vi "Process.vi"(8 "error in":errorcluster, 11 "SynchiIO.PXI4461":refnum<class "SynchiIO.PXI4461.lvclass">) -> (0 "error out":errorcluster, 3 "SynchiIO.PXI4461 out":refnum<class "SynchiIO.PXI4461.lvclass">)   [LabVIEW 2016, in "SynchiIO.PXI4461.lvclass"]
doc: "---------------------------------------------------------------\nJKI State Machine Objects™\nhttp://jki.net/state-machine-objects/\nCopyright (C) 2005-2015, JKI <info@jki.net>\nALL RIGHTS RESERVEDJKI State Machine Objects (SMO) 1.0.0.5\nJKI - JKI\nCopyright (c) 2016, JKI"
uses:
  SynchiIO.PXI4461.lvclass
  <vilib>/JKI/JKI SMO/SMO/SMO.lvclass
  <vilib>/JKI/JKI SMO/SMO/Typedefs/Parent Call--Enum.ctl
  <resource>/objmgr/ni.dex.rc
  trunk/SynchIO/SynchIO.USB4431/SynchIO.USB4431.lvclass
  C:/Program Files (x86)/National Instruments/LabVIEW 2016/vi.lib/JKI/JKI SMO/SMO/SMO.lvclass
  I:/levy_SVN/lockin/branches/jlevy/SMO/trunk/SynchIO/SynchIO/SynchIO.lvclass
panel:
  in  "Start":bool
  in  "stop":bool
  out "State History":string
  out "Current State":string="Exit"
  in  "Tab Control":T1(tab)=enum."AO Config"
  in  "AI Configuration":T2(array[cluster])=[{"AI.Coupling"=enum."DC", "AI.Max"=10.0, "AI.Min"=-10.0, "Input physical channels"="Dev1/ai0:3"}]
  in  "AO Configuration":T3(array[cluster])=[{"Output physical channels"="Dev1/ao0", "AO. Max"=3.5, "AO.Min"=-3.5}]
  in  "sampling info":cluster{"Fs":dbl, "#s":dbl}={"Fs"=102388.0, "#s"=7876.0}
  in  "AI Buffer Size (S)":i32=100
  in  "error in 2":errorcluster
  out "error out 2":errorcluster
  in  "AO":T4={"AO amp (V)"=[1.0, 0.0, 0.0, 0.0, 0.0, 0.0, 0.0, 0.0], "AO DC (V)"=[0.0, 0.0, 0.0, 0.0, 0.0, 0.0, 0.0, 0.0], "AO f (Hz)"=[13.0, 13.0, 13.0, 13.0, 13.0, 13.0, 13.0, 13.0], "AO phi (deg)"=[0.0, 0.0, 0.0, 0.0, 0.0, 0.0, 0.0, 0.0], "function"=[enum."Sine Wave", enum."Sine Wave", enum."Sine Wave", enum."Sine Wave", enum."Sine Wave", enum."Sine Wave", enum."Sine Wave", enum."Sine Wave"]} {"AO DC (V)" format="%#_6p"; "AO amp (V)" format="%#_6p"}
  out "Signals Graph":waveform(dbl)[](graph)=[{"t0"=timestamp(3565974471.4961195 s since 1904-01-01), "dt"=1.0, "Y"=array[6023 elements], "attributes"=variant("NI_ChannelName"=variant(string "Dev2/ai0"), "NI_UnitDescription"=variant(string "Volts"))}, {"t0"=timestamp(3565974471.4961195 s since 1904-01-01), "dt"=1.0, "Y"=array[6023 elements], "attributes"=variant("NI_ChannelName"=variant(string "Dev2/ai1"), "NI_UnitDescription"=variant(string "Volts"))}, {"t0"=timestamp(3565974471.4961195 s since 1904-01-01), "dt"=1.0, "Y"=array[6023 elements], "attributes"=variant("NI_ChannelName"=variant(string "Dev2/ai2"), "NI_UnitDescription"=variant(string "Volts"))}, {"t0"=timestamp(3565974471.4961195 s since 1904-01-01), "dt"=1.0, "Y"=array[6023 elements], "attributes"=variant("NI_ChannelName"=variant(string "Dev2/ai3"), "NI_UnitDescription"=variant(string "Volts"))}, {"t0"=timestamp(3565974471.554943 s since 1904-01-01), "dt"=1.0, "Y"=array[6023 elements], "attributes"=variant("NI_ChannelName"=variant(string "Dev2/ai0"), "NI_UnitDescription"=variant(string "Volts"))}, {"t0"=timestamp(3565974471.554943 s since 1904-01-01), "dt"=1.0, "Y"=array[6023 elements], "attributes"=variant("NI_ChannelName"=variant(string "Dev2/ai1"), "NI_UnitDescription"=variant(string "Volts"))}]
  out "Signals Graph 2":waveform(dbl)[](graph)=[{"t0"=timestamp(3565974471.4961195 s since 1904-01-01), "dt"=1.0, "Y"=array[6023 elements], "attributes"=variant("NI_ChannelName"=variant(string "Dev2/ai0"), "NI_UnitDescription"=variant(string "Volts"))}, {"t0"=timestamp(3565974471.4961195 s since 1904-01-01), "dt"=1.0, "Y"=array[6023 elements], "attributes"=variant("NI_ChannelName"=variant(string "Dev2/ai1"), "NI_UnitDescription"=variant(string "Volts"))}, {"t0"=timestamp(3565974471.4961195 s since 1904-01-01), "dt"=1.0, "Y"=array[6023 elements], "attributes"=variant("NI_ChannelName"=variant(string "Dev2/ai2"), "NI_UnitDescription"=variant(string "Volts"))}, {"t0"=timestamp(3565974471.4961195 s since 1904-01-01), "dt"=1.0, "Y"=array[6023 elements], "attributes"=variant("NI_ChannelName"=variant(string "Dev2/ai3"), "NI_UnitDescription"=variant(string "Volts"))}, {"t0"=timestamp(3565974471.554943 s since 1904-01-01), "dt"=1.0, "Y"=array[6023 elements], "attributes"=variant("NI_ChannelName"=variant(string "Dev2/ai0"), "NI_UnitDescription"=variant(string "Volts"))}, {"t0"=timestamp(3565974471.554943 s since 1904-01-01), "dt"=1.0, "Y"=array[6023 elements], "attributes"=variant("NI_ChannelName"=variant(string "Dev2/ai1"), "NI_UnitDescription"=variant(string "Volts"))}]
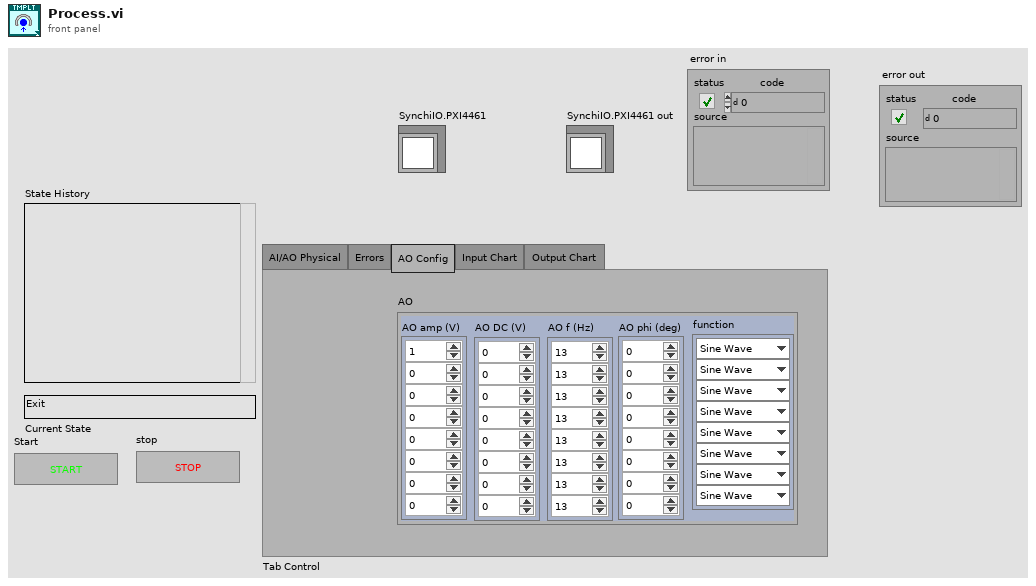
[diagram p1: front panel]
types:
  T1 = enum32{"AI/AO Physical", "Errors", "AO Config", "Input Chart", "Output Chart "}
  T2 = cluster{"AI.Coupling":enum16{"AC", "DC", "GND"}, "AI.Max":dbl, "AI.Min":dbl, "Input physical channels":tag}[]
  T3 = cluster{"Output physical channels":tag, "AO. Max":dbl, "AO.Min":dbl}[]
  T4 = cluster{"AO amp (V)":dbl[], "AO DC (V)":dbl[], "AO f (Hz)":dbl[], "AO phi (deg)":dbl[], "function":enum16{"Sine Wave", "Triangle Wave", "Square Wave", "Sawtooth Wave"}[]}
  T5 = typedef "SMO.lvclass/Parent Call--Enum.ctl" = enum16{"Allows parent to run", "Does not request parent to run"}
  T6 = enum32{"invalid app kind", "Development System", "Run Time System", "Student Edition", "Embedded LabVIEW", "Evaluation", "Custom"}
  T7 = enum32{"Invalid", "Standard", "Closed", "Hidden", "Minimized", "Maximized"}
  T8 = cluster{"Core":cluster{"Current VI Reference":refnum<vi>, "Close Panel on Exit?":bool, "error":errorcluster}, "Self Reference":refnum<class "SynchiIO.PXI4461.lvclass">, "Your string data":string, "AI Buffer Size (S)":i32, "AI Configuration":cluster{"AI.Coupling":enum16{"AC", "DC", "GND"}, "AI.Max":dbl, "AI.Min":dbl, "Input physical channels":tag}[], "AO Configuration":cluster{"Output physical channels":tag, "AO. Max":dbl, "AO.Min":dbl}[], "sampling info":cluster{"Fs":dbl, "#s":dbl}, "AI task":refnum<k21>[], "AO Task":refnum<k21>[], "AI Data":waveform(dbl)[], "AO Data":waveform(dbl)[], "AO":cluster{"AO amp (V)":dbl[], "AO DC (V)":dbl[], "AO f (Hz)":dbl[], "AO phi (deg)":dbl[], "function":enum16{"Sine Wave", "Triangle Wave", "Square Wave", "Sawtooth Wave"}[]}, "Iteration":i32, "writer endpoint":refnum<k21>, "reader endpoint":refnum<k21>, "url":string}
  T9 = cluster{"Current VI Reference":refnum<vi>, "Close Panel on Exit?":bool, "error":errorcluster}
  T10 = typedef "SynchIO.USB4431.lvclass/ProtectedEvents--Cluster.ctl" = cluster{"API_Template":refnum<user-event>}
  T11 = typedef "SynchiIO.PXI4461.lvclass/ProtectedEvents--Cluster.ctl" = cluster{"API_Template":refnum<user-event>}
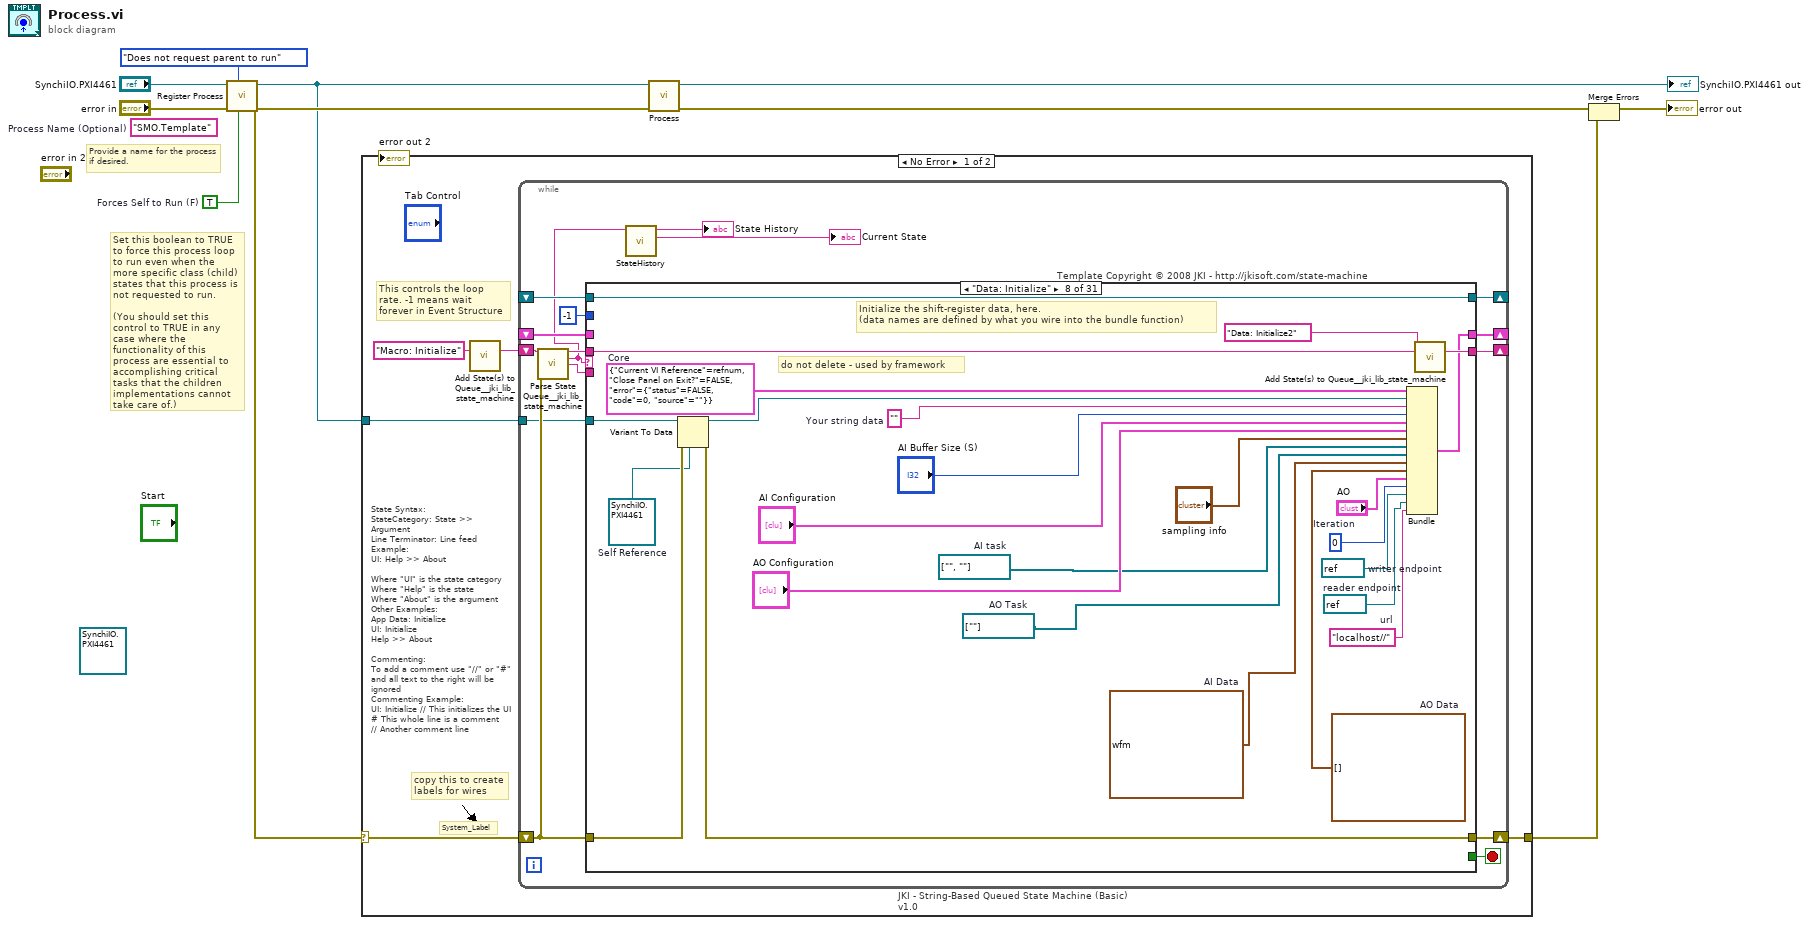
[diagram p0: block diagram]
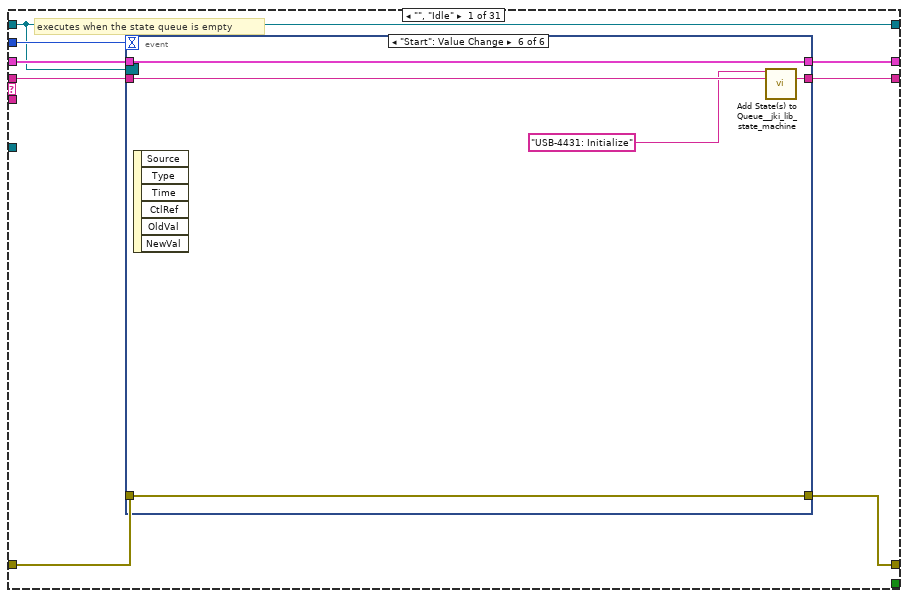
[diagram p2: hidden frame]
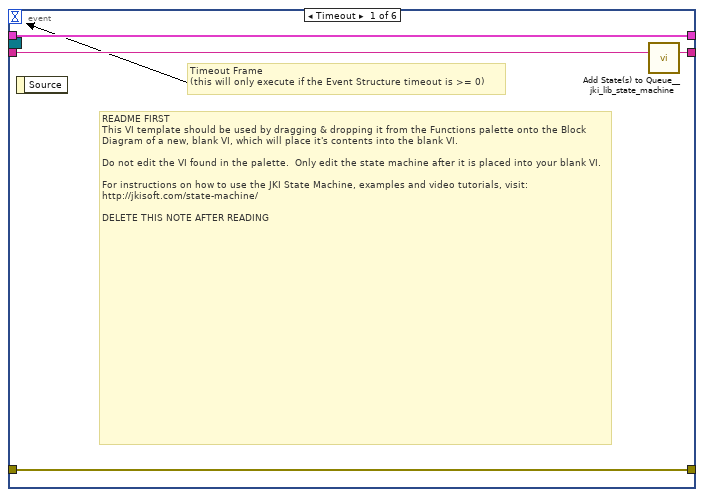
[diagram p3: hidden frame]
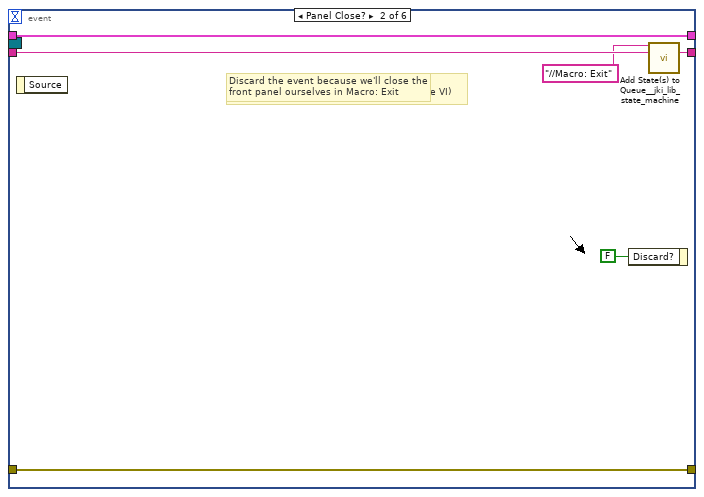
[diagram p4: hidden frame]
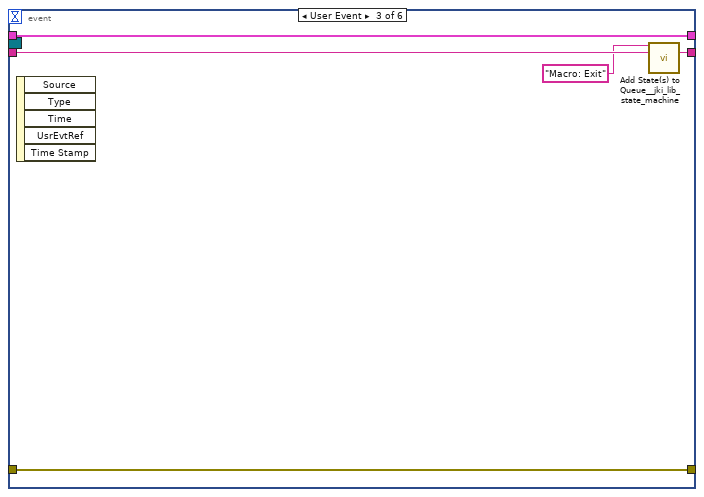
[diagram p5: hidden frame]
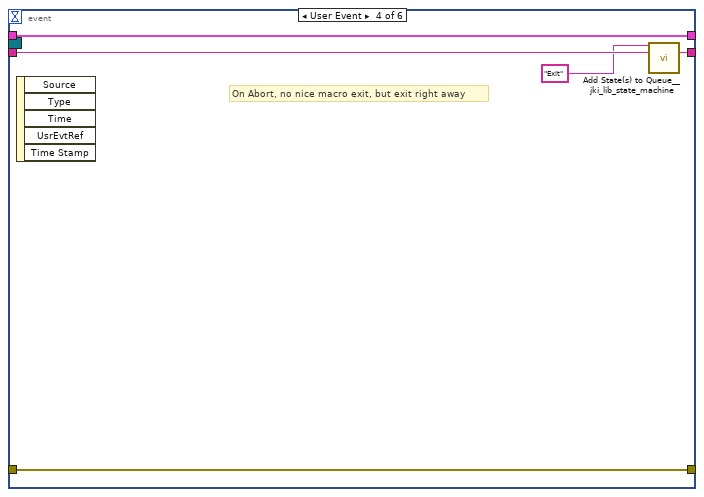
[diagram p6: hidden frame]
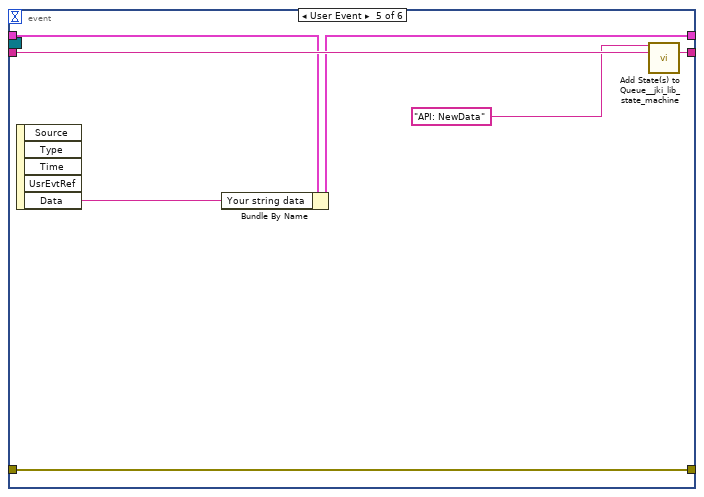
[diagram p7: hidden frame]
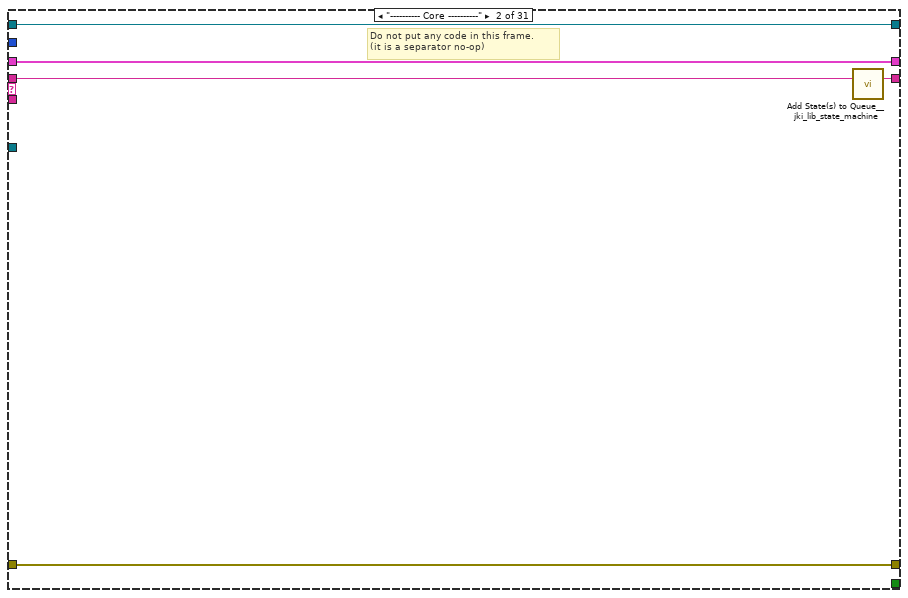
[diagram p8: hidden frame]
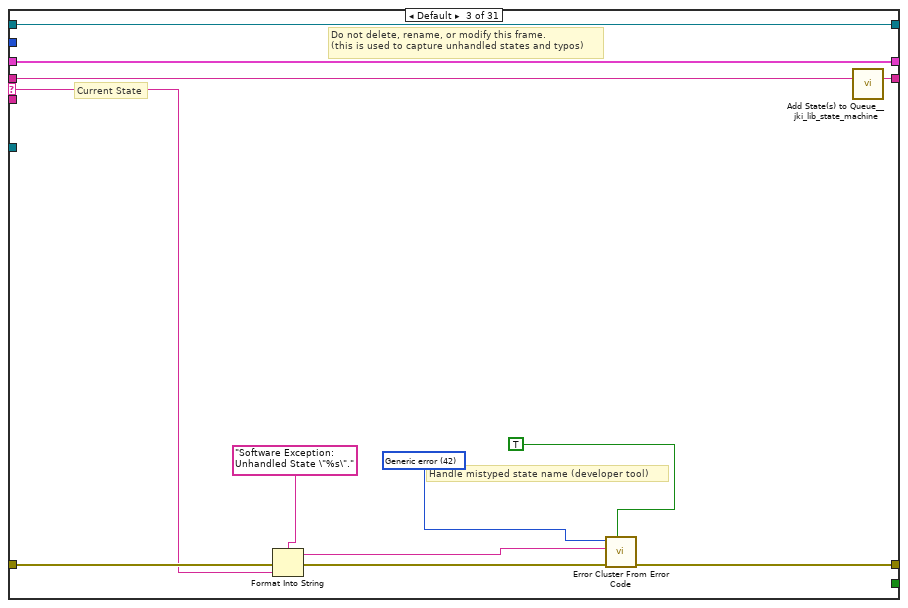
[diagram p9: hidden frame]
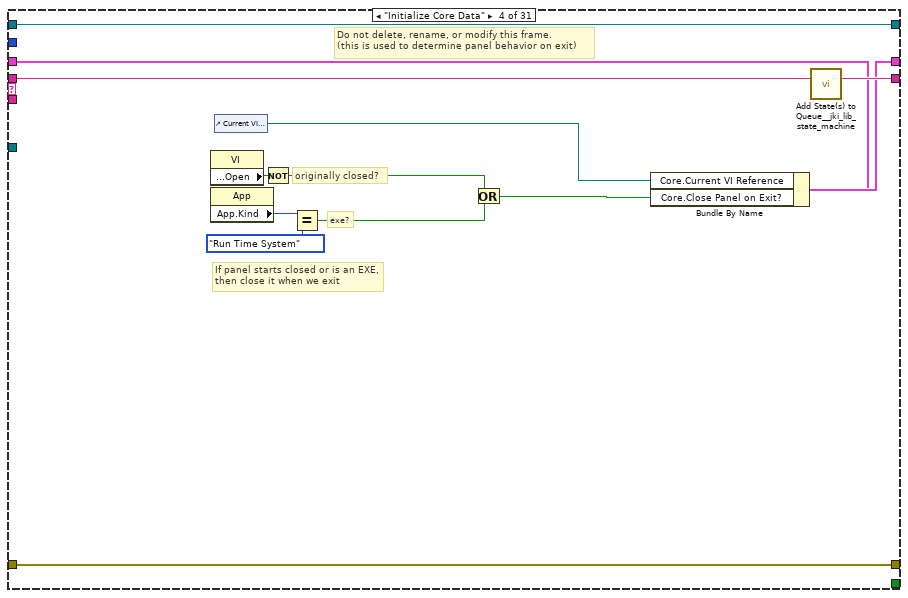
[diagram p10: hidden frame]
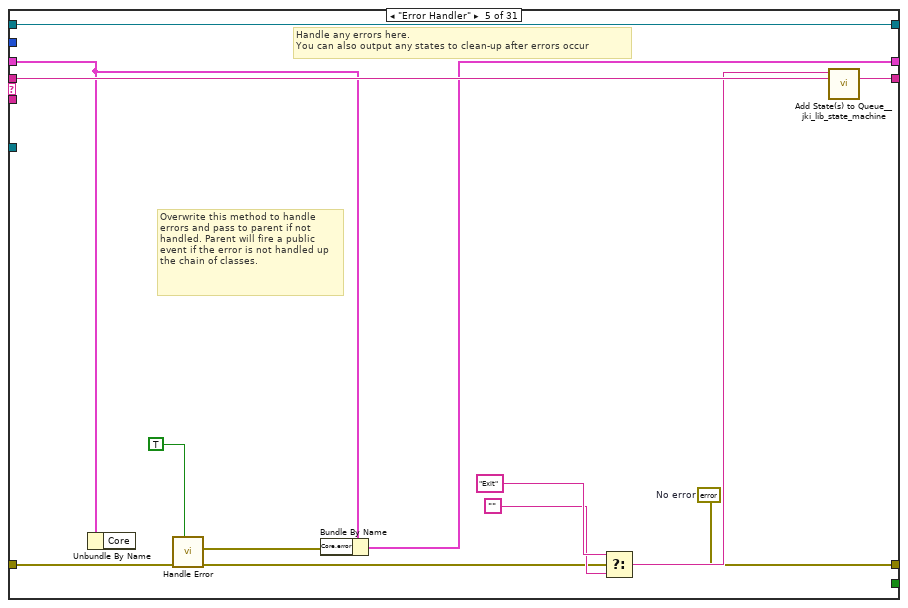
[diagram p11: hidden frame]
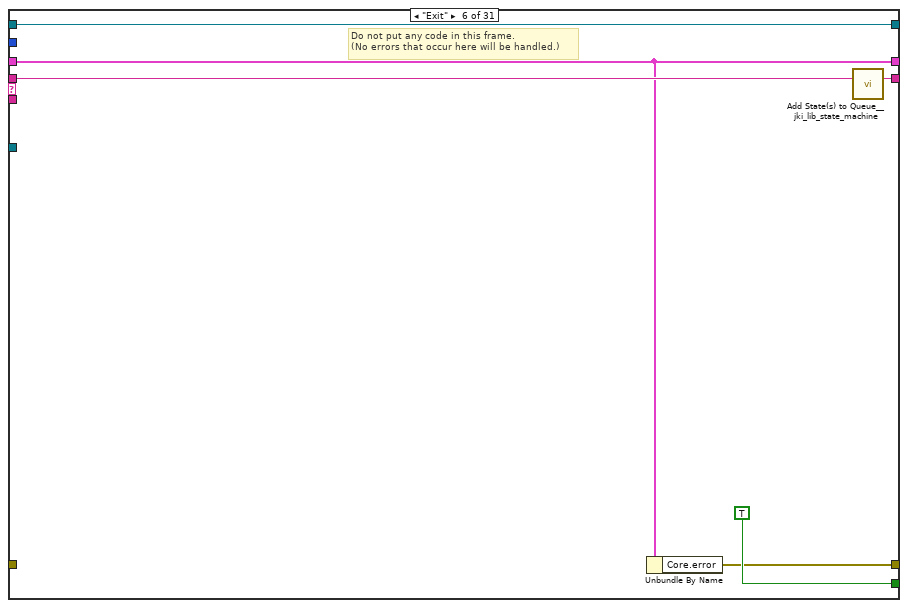
[diagram p12: hidden frame]
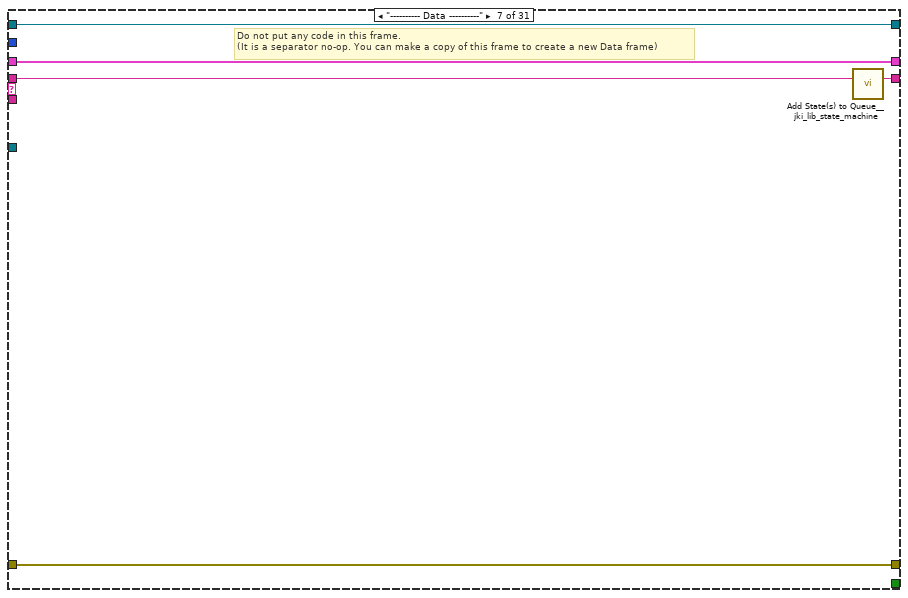
[diagram p13: hidden frame]
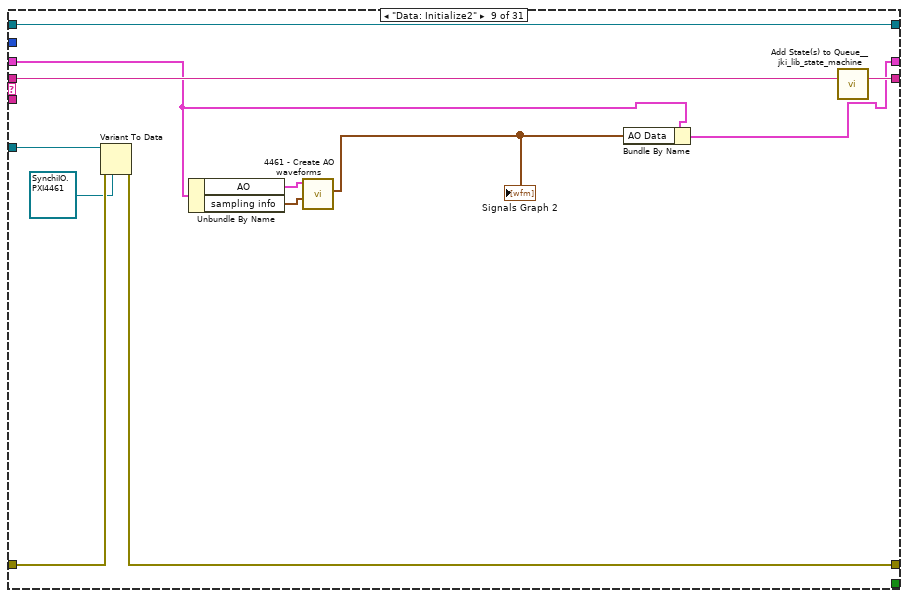
[diagram p14: hidden frame]
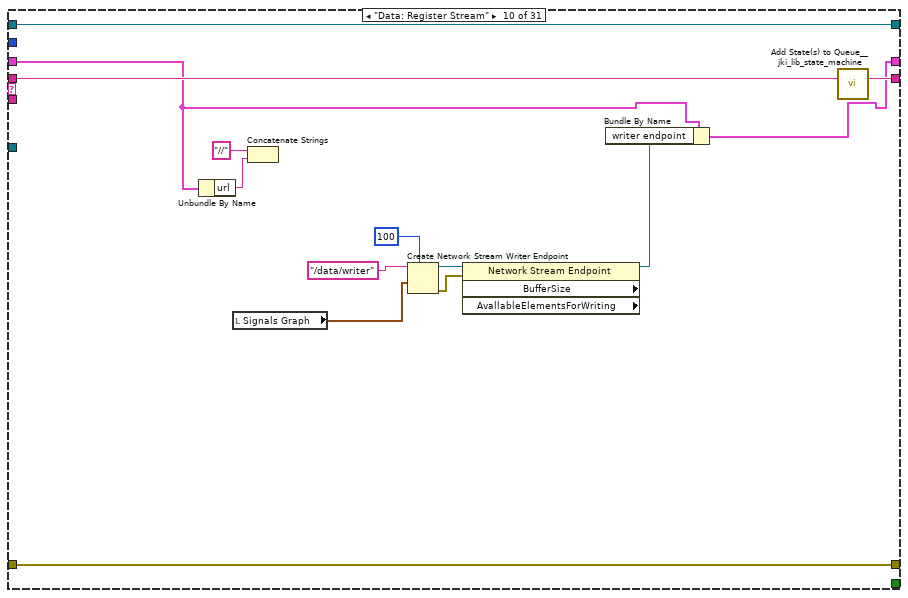
[diagram p15: hidden frame]
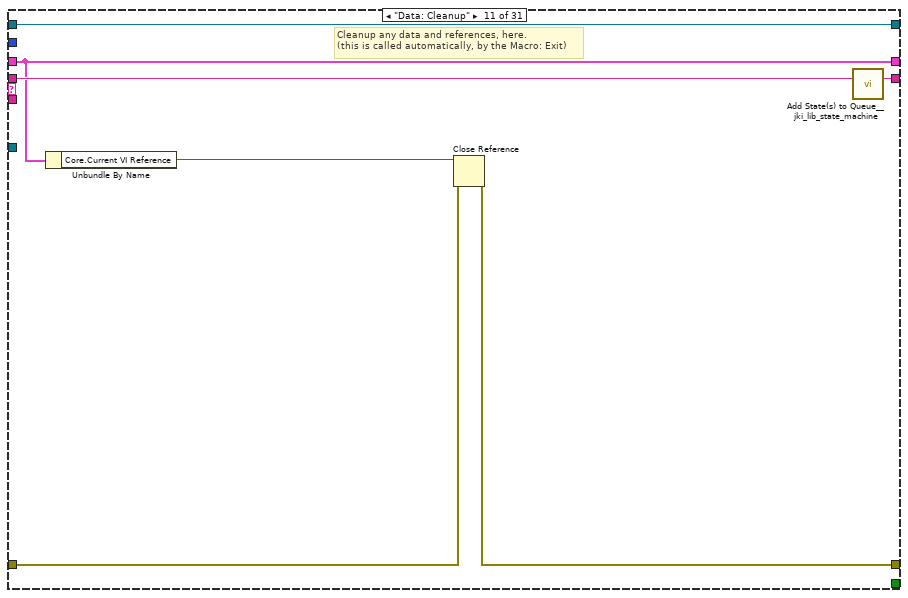
[diagram p16: hidden frame]
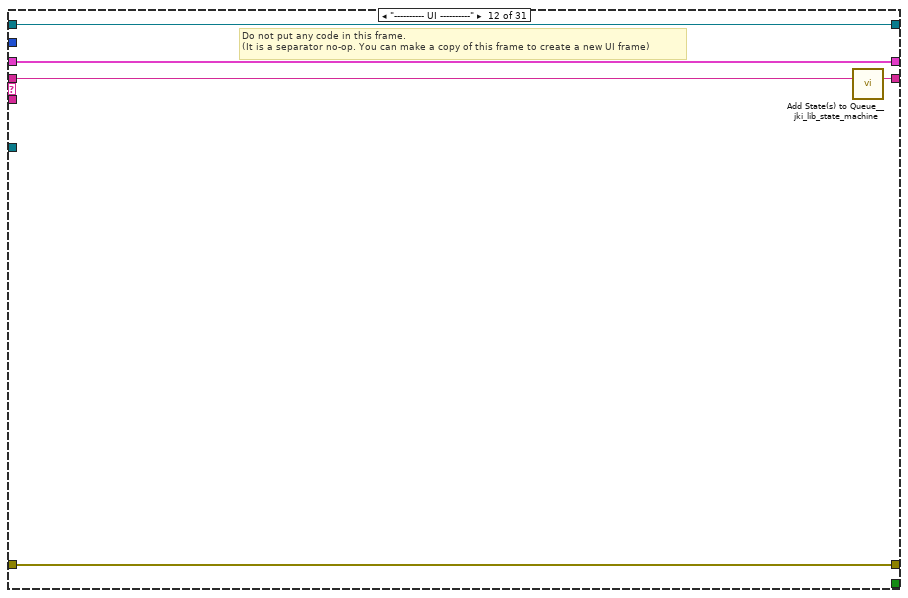
[diagram p17: hidden frame]
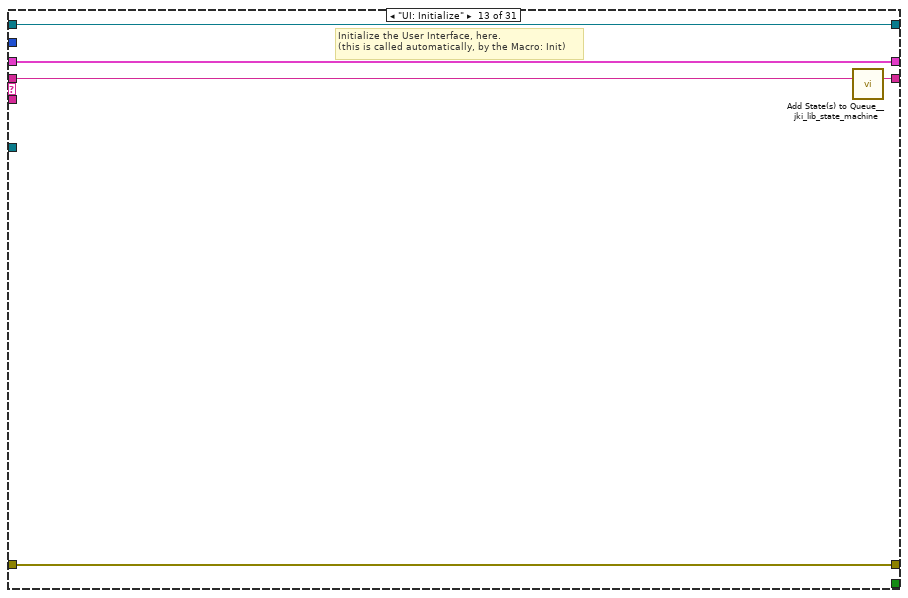
[diagram p18: hidden frame]
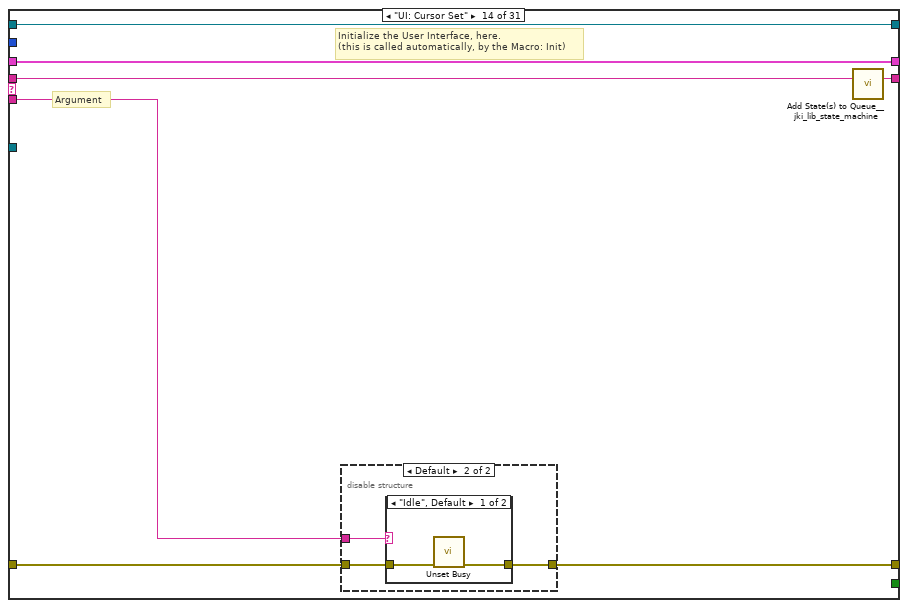
[diagram p19: hidden frame]
diagram:
  (unwired) refnum<class "SynchiIO.PXI4461.lvclass"> refnum ("SynchiIO.PXI4461.lvclass")
  w4 = TRUE  # Forces Self to Run (F)
  (unwired) "SMO.Template"  # Process Name (Optional)
  # "Provide a name for the process\nif desired."
  # "Set this boolean to TRUE to force this process loop to run even when the more specific class (child) states that this process is not requested to run.\n\n(You should set this control to TRUE in any case where the functionality of this process are essential to accomplishing critical tasks that the children implementations cannot take care of.)"
  n1 = call <vilib>:"Register Process.vi"("Forces Self to Run (F)"=w4, "Parent Call"=Parent_Call--Enum."Does not request parent to run", "error in (no error)"="error in", "SMO"="SynchiIO.PXI4461") -> ("error out"=w2:errorcluster, "SMO out"=w1:refnum<class "SynchiIO.PXI4461.lvclass">)  [unwired: 6 in]
  n2 = case shown="No Error" w2 {
    selector: w2 -> [w12 w407]
    tunnel: w1 -> [w13 _]
    tunnel: [w11 w407] -> w3
    frame No Error {
      # "State Syntax:\nStateCategory: State >> Argument\nLine Terminator: Line feed\nExample:\nUI: Help >> About\n\nWhere \"UI\" is the state category\nWhere \"Help\" is the state\nWhere \"About\" is the argument\nOther Examples:\nApp Data: Initialize\nUI: Initialize\nHelp >> About\n\nCommenting:\nTo add a comment use \"//\" or \"#\" and all text to the right will be ignored\nCommenting Example:\nUI: Initialize // This initializes the UI\n# This whole line is a comment\n// Another comment line"
      # "copy this to create labels for wires"
      # "This controls the loop rate. -1 means wait forever in Event Structure"
      # "System_Label"
      n3 = call <vilib>:"Add State(s) to Queue__jki_lib_state_machine.vi"("State(s) in (\"\")"="Macro: Initialize") -> ("States Out"=w15:string)  [unwired: 14 in]
      n4 = while "JKI - String-Based Queued State Machine (Basic) v1.0" {
        shift-right: [w26] -> _
        shift-left: _ -> [w25]
        shift-right: [w29] -> w11
        shift-left: w12 -> [w23]
        shift-right: [w28] -> _
        shift-left: w15 -> [w30]
        tunnel: w13 -> [w22]
        shift-right: [w21] -> _
        shift-left: _ -> [w20]
        stop <- w27 stop-if-true
        # "Template Copyright © 2008 JKI - http://jkisoft.com/state-machine"
        n5 = call <vilib>:"Parse State Queue__jki_lib_state_machine.vi"("State Queue"=w30, "Error In (no error)"=w23) -> ("Remaining States"=w17:string, "Current State"=w16:string, "Arguments"=w31:string)  [unwired: 11 in]
        n6 = case shown="\"Data: Initialize\"" w16 {
          selector: w16 -> [_ _ w78 _ _ _ _ _ _ _ _ _ _ _ _ _ _ _ _ _ _ _ _ _ _ _ _ _ _ _ _]
          tunnel: w17 -> [w39 w76 w82 w101 w114 w120 w125 w150 w162 w176 w183 w188 w193 w200 w216 w248 w257 w271 w276 w287 w296 w308 w314 w319 w326 w331 w336 w352 w369 w381 w393]
          tunnel: w31 -> [_ _ _ _ _ _ _ _ _ _ _ _ _ w194 w210 _ _ _ _ _ _ _ _ _ _ _ _ _ _ _ _]
          tunnel: w25 -> [w37 w73 w80 w92 w104 w116 w122 _ w154 w173 w178 w185 w191 w198 w212 w245 w253 w262 w273 w284 w293 w306 w312 w317 w323 w328 w334 w345 w366 w378 w388]
          tunnel: [w36 w74 w84 w98 w106 w115 w123 w145 w159 w166 w179 w186 w190 w195 w213 w246 w255 w269 w274 w278 w294 w301 w310 w315 w321 w327 w332 w341 w361 w375 w390] -> w29
          tunnel: w23 -> [w35 w74 w83 w98 w111 _ w123 w146 w160 w166 w180 w186 w190 w196 w214 w246 w255 w269 w274 w279 w294 w303 w310 w315 w322 w327 w332 w342 w356 w375 w389]
          tunnel: [w38 w75 w81 w100 w113 w119 w124 w149 w161 w175 w182 w187 w192 w199 w215 w247 w256 w270 w275 w286 w295 w307 w313 w318 w325 w330 w335 w351 w368 w380 w392] -> w28
          tunnel: [_ _ _ _ _ TRUE _ _ _ _ _ _ _ _ _ _ _ _ _ _ _ _ _ _ _ _ _ _ _ _ _] -> w27
          tunnel: [w34 w73 w80 w99 w103 w116 w122 w148 w153 w172 w178 w185 w191 w198 w212 w245 w253 w262 w273 w284 w293 w306 w312 w317 w323 w328 w334 w344 w365 w377 w388] -> w26
          tunnel: -1 ("Timeout") -> [w33 _ _ _ _ _ _ _ _ _ _ _ _ _ _ _ _ _ _ _ _ _ _ _ _ _ _ _ _ _ _]
          tunnel: w22 -> [_ _ _ _ _ _ _ w144 w158 _ _ _ _ _ _ _ _ _ _ _ _ _ _ _ _ _ _ _ _ _ _]
          tunnel: [w32 w72 w77 w89 w112 w117 w121 w142 w157 w174 w177 w184 w189 w197 w209 w244 w254 w263 w272 w285 w292 w305 w311 w316 w324 w329 w333 w350 w367 w379 w391] -> w21
          tunnel: w20 -> [w32 w72 w77 w89 w112 w117 w121 w142 w157 w174 w177 w184 w189 w197 w209 w244 w254 w263 w272 w285 w292 _ w311 w316 w324 w329 w333 w350 w367 w379 w391]
          frame "", "Idle" {
            # "executes when the state queue is empty"
            n7 = event shown="[5] \"Start\": Value Change" {
              selector: w32 -> [_ _ _ _ _ _]
              dyn-events: _ -> [_ _ _ _ _ _]
              timeout: w33 -> [_ _ _ _ _ _]
              tunnel: w39 -> [w43 w49 w54 w59 w66 w71]
              tunnel: [w42 w48 w53 w58 w65 w70] -> w38
              tunnel: w37 -> [w40 w46 w51 w56 w63 w67]
              tunnel: [w41 w47 w52 w57 w64 w69] -> w36
              tunnel: w35 -> [w41 w47 w52 w57 w64 w69]
              tunnel: [w40 w46 w51 w56 w62 w67] -> w34
              event Timeout {
                # "README FIRST\nThis VI template should be used by dragging & dropping it from the Functions palette onto the Block Diagram of a new, blank VI, which will place it's contents into the blank VI.\n\nDo not edit the VI found in the palette.  Only edit the state machine after it is placed into your blank VI.\n\nFor instructions on how to use the JKI State Machine, examples and video tutorials, visit:\nhttp://jkisoft.com/state-machine/\n\nDELETE THIS NOTE AFTER READING"
                # "Timeout Frame\n(this will only execute if the Event Structure timeout is >= 0)"
                n8 = event-data() -> ()  [unwired: 1 in, 1 out]
                n9 = call <vilib>:"Add State(s) to Queue__jki_lib_state_machine.vi"("State(s) in (\"\")"=w43) -> ("States Out"=w42:string)  [unwired: 14 in]
              }
              event Panel Close? {
                # "Discard the event because we'll close the front panel ourselves in Macro: Exit"
                # "Close Panel button (pressed) Event\n(this executes Macro: Exit to terminate the VI)"
                n10 = event-data() -> ()  [unwired: 1 in, 1 out]
                n11 = event-data("Discard?"=FALSE) -> ()  [unwired: 1 in, 1 out]
                n12 = call <vilib>:"Add State(s) to Queue__jki_lib_state_machine.vi"("State(s) in Front (\"\")"="//Macro: Exit", "State(s) in (\"\")"=w49) -> ("States Out"=w48:string)  [unwired: 13 in]
              }
              event User Event {
                n13 = event-data() -> ()  [unwired: 1 in, 5 out]
                n14 = call <vilib>:"Add State(s) to Queue__jki_lib_state_machine.vi"("State(s) in Front (\"\")"="Macro: Exit", "State(s) in (\"\")"=w54) -> ("States Out"=w53:string)  [unwired: 13 in]
              }
              event User Event {
                # "On Abort, no nice macro exit, but exit right away"
                n15 = event-data() -> ()  [unwired: 1 in, 5 out]
                n16 = call <vilib>:"Add State(s) to Queue__jki_lib_state_machine.vi"("State(s) in Front (\"\")"="Exit", "State(s) in (\"\")"=w59) -> ("States Out"=w58:string)  [unwired: 13 in]
              }
              event User Event {
                n17 = event-data() -> ("Data"=w60:string)  [unwired: 1 in, 4 out]
                n18 = Bundle By Name(cluster=w63, "Your string data"=w60) -> (w62:T8)
                n19 = call <vilib>:"Add State(s) to Queue__jki_lib_state_machine.vi"("State(s) in Front (\"\")"="API: NewData", "State(s) in (\"\")"=w66) -> ("States Out"=w65:string)  [unwired: 13 in]
              }
              event "Start": Value Change {
                n20 = event-data() -> ()  [unwired: 1 in, 6 out]
                n21 = call <vilib>:"Add State(s) to Queue__jki_lib_state_machine.vi"("State(s) in Front (\"\")"="USB-4431: Initialize", "State(s) in (\"\")"=w71) -> ("States Out"=w70:string)  [unwired: 13 in]
              }
            }
          }
          frame "---------- Core ----------" {
            # "Do not put any code in this frame.\n(it is a separator no-op)"
            n22 = call <vilib>:"Add State(s) to Queue__jki_lib_state_machine.vi"("State(s) in (\"\")"=w76) -> ("States Out"=w75:string)  [unwired: 14 in]
          }
          frame Default {
            w87 = 42 items=["No error", "Argument error", "Memory is full", "Out of zone", "End of file", "File already open", "Generic file I/O error", "File not found", "File permission error", "Disk is full", "Duplicate path", "Too many files open", "System feature not enabled", "Resource file not found", "Cannot add resource", "Resource not found", "Image not found", "Image memory error", "Pen does not exist", "Config type invalid", "Config token not found", "Config parse error", "Config memory error", "Bad external code format", "Bad external code offset", "External code not present", "Null window", "Destroy window error", "Null menu", "Print aborted", "Bad print record", "Print driver error", "Windows error during printing", "Memory error during printing", "Print dialog error", "Generic print error", "Invalid device refnum", "Device not found", "Device parameter error", "Device unit error", "Cannot open device", "Device call aborted", "Generic error", "Cancelled by user", "Object ID too low", "Object ID too high", "Object not in heap", "Unknown heap", "Unknown object (invalid DefProc)", "Unknown object (DefProc not in table)", "Message out of range", "Invalid (null) method", "Unknown message", "Manager call not supported", "Bad address", "Network operation in progress", "Network operation timed out", "Connection is busy", "Network attribute not supported", "Network error", "Address in use", "System out of memory", "Connection aborted", "Connection refused", "Not connected", "Already connected", "Connection closed", "Initialization error (interapplication manager)", "Bad occurrence", "Wait on unbound occurrence handler", "Occurrence queue overflow", "Datalog type conflict", "Unused", "Unrecognized type (interapplication manager)", "Memory corrupt", "Failed to make temporary DLL", "Old CIN version", "Drag socket not found", "Failed to load drop-object", "Failed to register OLE object", "Failed to release OLE object", "Format specifier type mismatch", "Unknown format specifier", "Too few format specifiers", "Too many format specifiers", "Scan failed", "Newer CIN version", "Error converting to variant", "Runtime menu error", "Password tampered", "Variant attribute not found", "Incompatible variant data type", "Event data is not available", "Event Store is not present", "Occurrence is not found", "Event Queue is not created", "Event info is not available", "Refnum passed is NULL", "Error retrieving Class GUID", "Error retrieving CoClass GUID", "Error retrieving TypeLib GUID.", "Bad built application magic bytes.", "Specific driver is different from the specific driver associated with the Logical Name.", "There is no session opened to the class driver.", "Max Error", "MAX - Error with config objects", "MAX - Error loading configuration", "MAX - Group not supported"]
            # "Current State"
            # "Do not delete, rename, or modify this frame.\n(this is used to capture unhandled states and typos)"
            # "Handle mistyped state name (developer tool)"
            n23 = Format Into String(format string="Software Exception: Unhandled State \"%s\"." ("message"), error in=w83, w78) -> (resulting string=w86:string, error out=w85:errorcluster)  [unwired: 1 in]
            n24 = call <vilib>:"Error Cluster From Error Code.vi"("show call chain? (False)"=TRUE, "error in (no error)"=w85, "error message (\"\")"=w86, "error code (0)"=w87) -> ("error out"=w84:errorcluster)  [unwired: 5 in]
            n25 = call <vilib>:"Add State(s) to Queue__jki_lib_state_machine.vi"("State(s) in (\"\")"=w82) -> ("States Out"=w81:string)  [unwired: 14 in]
          }
          frame "Initialize Core Data" {
            # "Do not delete, rename, or modify this frame.\n(this is used to determine panel behavior on exit)"
            # "originally closed?"
            # "exe?"
            # "If panel starts closed or is an EXE, then close it when we exit"
            n26 = property class="VI"() -> ("Front Panel.Open"=w97:bool)  [unwired: 2 in, 2 out]
            n27 = property class="App"() -> ("App.Kind"=w96:T6)  [unwired: 2 in, 2 out]
            n28 = control-ref of="Current VI Reference"() -> (w90:refnum<vi>)
            n29 = Not(x=w97) -> (.not. x?=w94:bool)
            n30 = Equal?(x=w96, y=T6."Run Time System" ("Application:Kind")) -> (x = y?=w93:bool)
            n31 = Or(x=w94, y=w93) -> (x .or. y?=w91:bool)
            n32 = Bundle By Name(cluster=w92, "Core.Current VI Reference"=w90, "Core.Close Panel on Exit?"=w91) -> (w99:T8)
            n33 = call <vilib>:"Add State(s) to Queue__jki_lib_state_machine.vi"("State(s) in (\"\")"=w101) -> ("States Out"=w100:string)  [unwired: 14 in]
          }
          frame "Error Handler" {
            w106 = errorcluster {"status"=FALSE, "code"=0, "source"=""}  # No error
            # "Overwrite this method to handle errors and pass to parent if not handled. Parent will fire a public event if the error is not handled up the chain of classes."
            # "Handle any errors here.\nYou can also output any states to clean-up after errors occur"
            n34 = Unbundle By Name(w104) -> ()  [unwired: 1 out]
            n35 = call-dynamic "Handle Error.vi"("Stop on Unhandled Error (T)"=TRUE, "error in"=w111) -> ("handling error"=w107:errorcluster, "Unhandled error"=w105:errorcluster)  [unwired: 7 in, 1 out]
            n36 = Bundle By Name(cluster=w104, "Core.error"=w105) -> (w103:T8)
            n37 = Select(t="Exit", s=w107, f="") -> (s? t:f=w108:string)
            n38 = call <vilib>:"Add State(s) to Queue__jki_lib_state_machine.vi"("State(s) in Front (\"\")"=w108, "State(s) in (\"\")"=w114) -> ("States Out"=w113:string)  [unwired: 13 in]
          }
          frame "Exit" {
            # "Do not put any code in this frame.\n(No errors that occur here will be handled.)"
            n39 = Unbundle By Name(w116) -> ("Core.error"=w115:errorcluster)
            n40 = call <vilib>:"Add State(s) to Queue__jki_lib_state_machine.vi"("State(s) in (\"\")"=w120) -> ("States Out"=w119:string)  [unwired: 14 in]
          }
          frame "---------- Data ----------" {
            # "Do not put any code in this frame.\n(It is a separator no-op. You can make a copy of this frame to create a new Data frame)"
            n41 = call <vilib>:"Add State(s) to Queue__jki_lib_state_machine.vi"("State(s) in (\"\")"=w125) -> ("States Out"=w124:string)  [unwired: 14 in]
          }
          frame "Data: Initialize" {
            w126 = refnum<class "SynchiIO.PXI4461.lvclass"> refnum  # Self Reference
            w127 = "localhost//"  # url
            w128 = refnum<k21> refnum  # reader endpoint
            w129 = waveform(dbl)[] [{"t0"=timestamp(3565974471.4961195 s since 1904-01-01), "dt"=1.0, "Y"=array[6023 elements], "attributes"=variant("NI_ChannelName"=variant(string "Dev2/ai0"), "NI_UnitDescription"=variant(string "Volts"))}, {"t0"=timestamp(3565974471.4961195 s since 1904-01-01), "dt"=1.0, "Y"=array[6023 elements], "attributes"=variant("NI_ChannelName"=variant(string "Dev2/ai1"), "NI_UnitDescription"=variant(string "Volts"))}, {"t0"=timestamp(3565974471.4961195 s since 1904-01-01), "dt"=1.0, "Y"=array[6023 elements], "attributes"=variant("NI_ChannelName"=variant(string "Dev2/ai2"), "NI_UnitDescription"=variant(string "Volts"))}, {"t0"=timestamp(3565974471.4961195 s since 1904-01-01), "dt"=1.0, "Y"=array[6023 elements], "attributes"=variant("NI_ChannelName"=variant(string "Dev2/ai3"), "NI_UnitDescription"=variant(string "Volts"))}, {"t0"=timestamp(3565974471.554943 s since 1904-01-01), "dt"=1.0, "Y"=array[6023 elements], "attributes"=variant("NI_ChannelName"=variant(string "Dev2/ai0"), "NI_UnitDescription"=variant(string "Volts"))}, {"t0"=timestamp(3565974471.554943 s since 1904-01-01), "dt"=1.0, "Y"=array[6023 elements], "attributes"=variant("NI_ChannelName"=variant(string "Dev2/ai1"), "NI_UnitDescription"=variant(string "Volts"))}]  # AI Data
            w130 = refnum<k21> refnum  # writer endpoint
            w131 = 0  # Iteration
            w133 = waveform(dbl)[] []  # AO Data
            w134 = refnum<k21>[] [""]  # AO Task
            w135 = refnum<k21>[] ["", ""]  # AI task
            w141 = T9 {"Current VI Reference"=refnum, "Close Panel on Exit?"=FALSE, "error"={"status"=FALSE, "code"=0, "source"=""}}  # Core
            w147 = ""  # Your string data
            # "do not delete - used by framework"
            # "Initialize the shift-register data, here.\n(data names are defined by what you wire into the bundle function)"
            n42 = Variant To Data(error in=w146, type=w126, Variant=w144) -> (data=w143:refnum<class "SynchiIO.PXI4461.lvclass">, error out=w145:errorcluster)
            n43 = Bundle("Core"=w141, "Self Reference"=w143, "Your string data"=w147, "AI Buffer Size (S)"="AI Buffer Size (S)", "AI Configuration"="AI Configuration", "AO Configuration"="AO Configuration", "sampling info"="sampling info", "AI task"=w135, "AO Task"=w134, "AI Data"=w129, "AO Data"=w133, "AO"="AO", "Iteration"=w131, "writer endpoint"=w130, "reader endpoint"=w128, "url"=w127) -> (w148:T8)  [unwired: 1 in]
            n44 = call <vilib>:"Add State(s) to Queue__jki_lib_state_machine.vi"("State(s) in Front (\"\")"="Data: Initialize2" ("State(s) in Front (\"\")"), "State(s) in (\"\")"=w150) -> ("States Out"=w149:string)  [unwired: 13 in]
          }
          frame "Data: Initialize2" {
            n45 = Variant To Data(error in=w160, type=refnum<class "SynchiIO.PXI4461.lvclass"> refnum ("SynchiIO.PXI4461.lvclass"), Variant=w158) -> (error out=w159:errorcluster)  [unwired: 1 out]
            n46 = Unbundle By Name(w154) -> ("AO"=w155:T4, "sampling info"=w156:cluster{"Fs":dbl, "#s":dbl})
            n47 = call "4461 - Create AO waveforms.vi"("sampling info"=w156, "AO"=w155) -> ("AO Array"=w152:waveform(dbl)[])  [unwired: 6 in, 3 out]
            "Signals Graph 2" <- w152
            n48 = Bundle By Name(cluster=w154, "AO Data"=w152) -> (w153:T8)
            n49 = call <vilib>:"Add State(s) to Queue__jki_lib_state_machine.vi"("State(s) in (\"\")"=w162) -> ("States Out"=w161:string)  [unwired: 14 in]
          }
          frame "Data: Register Stream" {
            n50 = Unbundle By Name(w173) -> ("url"=w163:string)
            n51 = local read "Signals Graph"() -> (w165:waveform(dbl)[])
            n52 = Concatenate Strings("//" ("reader url"), w163) -> ()  [unwired: 1 out]
            n53 = Create Network Stream Writer Endpoint(7:100 ("writer buffer size"), 9:w165, 11:"/data/writer" ("reader url")) -> (0:w169:errorcluster, 3:w170:refnum<k21>)  [unwired: 4 in]
            n54 = property class="Network Stream Endpoint" props=["BufferSize", "AvallableElementsForWriting"](reference=w170, error in=w169) -> (reference out=w167:refnum<k21>)  [unwired: 3 out]
            n55 = Bundle By Name(cluster=w173, "writer endpoint"=w167) -> (w172:T8)
            n56 = call <vilib>:"Add State(s) to Queue__jki_lib_state_machine.vi"("State(s) in (\"\")"=w176) -> ("States Out"=w175:string)  [unwired: 14 in]
          }
          frame "Data: Cleanup" {
            # "Cleanup any data and references, here.\n(this is called automatically, by the Macro: Exit)"
            n57 = Unbundle By Name(w178) -> ("Core.Current VI Reference"=w181:refnum<vi>)
            n58 = Close Reference(reference=w181, error in (no error)=w180) -> (error out=w179:errorcluster)
            n59 = call <vilib>:"Add State(s) to Queue__jki_lib_state_machine.vi"("State(s) in (\"\")"=w183) -> ("States Out"=w182:string)  [unwired: 14 in]
          }
          frame "---------- UI ----------" {
            # "Do not put any code in this frame.\n(It is a separator no-op. You can make a copy of this frame to create a new UI frame)"
            n60 = call <vilib>:"Add State(s) to Queue__jki_lib_state_machine.vi"("State(s) in (\"\")"=w188) -> ("States Out"=w187:string)  [unwired: 14 in]
          }
          frame "UI: Initialize" {
            # "Initialize the User Interface, here.\n(this is called automatically, by the Macro: Init)"
            n61 = call <vilib>:"Add State(s) to Queue__jki_lib_state_machine.vi"("State(s) in (\"\")"=w193) -> ("States Out"=w192:string)  [unwired: 14 in]
          }
          frame "UI: Cursor Set" {
            # "Argument"
            # "Initialize the User Interface, here.\n(this is called automatically, by the Macro: Init)"
            n62 = disable-structure shown="Default" {
              disable-tunnel: w196 -> [w201 w204]
              disable-tunnel: [w201 w203] -> w195
              disable-tunnel: w194 -> [_ w202]
              frame condition #0 {
              }
              frame condition #1 (active) {
                n63 = case shown="\"Idle\", Default" w202 {
                  tunnel: w204 -> [w206 w208]
                  tunnel: [w205 w207] -> w203
                  frame "Idle", Default {
                    n64 = call <vilib>:"Unset Busy.vi"("error in (no error)"=w206) -> ("error out"=w205:errorcluster)  [unwired: 10 in]
                  }
                  frame "Busy" {
                    n65 = call <vilib>:"Set Busy.vi"("error in (no error)"=w208) -> ("error out"=w207:errorcluster)  [unwired: 9 in, 1 out]
                  }
                }
              }
            }
            n66 = call <vilib>:"Add State(s) to Queue__jki_lib_state_machine.vi"("State(s) in (\"\")"=w200) -> ("States Out"=w199:string)  [unwired: 14 in]
          }
          frame "UI: Front Panel State" {
            # "Argument"
            # "Set Front Panel Open or Closed\n(Usage: \"UI: Front Panel State >> Open|Close\")"
            n67 = Unbundle By Name(w212) -> ("Core.Current VI Reference"=w211:refnum<vi>)
            n68 = disable-structure shown="Default" {
              disable-tunnel: w214 -> [w220 w243]
              disable-tunnel: [w219 w243] -> w213
              disable-tunnel: w211 -> [w218 _]
              disable-tunnel: w210 -> [w217 _]
              frame condition #0 (active) {
                n69 = case shown="\"Open\", Default" w217 {
                  tunnel: w220 -> [w224 w237]
                  tunnel: [w226 w238] -> w219
                  tunnel: w218 -> [w225 w235]
                  frame "Open", Default {
                    n70 = property class="VI"(reference=w225, error in=w224) -> (reference out=w222:refnum<vi>, error out=w223:errorcluster, "FP.State"=w221:T7)
                    n71 = case shown="\"Closed\"" w221 {
                      tunnel: [w229 w232] -> w226
                      tunnel: w223 -> [w228 w232]
                      tunnel: w222 -> [w227 _]
                      frame "Closed" {
                        n72 = invoke class="VI" method="FP.Open"(reference=w227, error in=w228, "Activate"=TRUE, "State"=T7."Standard") -> (error out=w229:errorcluster)  [unwired: 1 in, 4 out]
                      }
                      frame Default {
                      }
                    }
                  }
                  frame "Close" {
                    n73 = property class="VI"(reference=w235, error in=w237) -> (reference out=w234:refnum<vi>, error out=w236:errorcluster, "FP.State"=w233:T7)
                    n74 = case shown="Default" w233 {
                      tunnel: [w239 w242] -> w238
                      tunnel: w236 -> [w239 w241]
                      tunnel: w234 -> [_ w240]
                      frame "Invalid", "Closed" {
                      }
                      frame Default {
                        n75 = invoke class="VI" method="FP.Close"(reference=w240, error in=w241) -> (error out=w242:errorcluster)  [unwired: 1 in, 2 out]
                      }
                    }
                  }
                }
              }
              frame condition #1 {
              }
            }
            n76 = call <vilib>:"Add State(s) to Queue__jki_lib_state_machine.vi"("State(s) in (\"\")"=w216) -> ("States Out"=w215:string)  [unwired: 14 in]
          }
          frame "---------- Macro ----------" {
            # "Do not put any code in this frame.\n(It is a separator no-op. You can make a copy of this frame to create a new Macro frame)"
            n77 = call <vilib>:"Add State(s) to Queue__jki_lib_state_machine.vi"("State(s) in (\"\")"=w248) -> ("States Out"=w247:string)  [unwired: 14 in]
          }
          frame "Macro: Initialize" {
            # "Initialization Macro\n(This is called once, when the VI starts)"
            n78 = call <vilib>:"Add State(s) to Queue__jki_lib_state_machine.vi"("State(s) in Front (\"\")"="Data: Initialize\nInitialize Core Data\nEvents: Register", "State(s) in (\"\")"="Process: Sync", "State(s) at Back (\"\")"="UI: Initialize\nUI: Front Panel State >> Open\nData: Register Stream") -> ("States Out"=w250:string)  [unwired: 12 in]
            n79 = call <vilib>:"Add State(s) to Queue__jki_lib_state_machine.vi"("State(s) in Front (\"\")"=w250, "State(s) in (\"\")"=w257) -> ("States Out"=w256:string)  [unwired: 13 in]
          }
          frame "Macro: Exit" {
            # "Exit Macro\n(This is called once, when the VI exits)"
            n80 = Unbundle By Name(w262) -> ("Core.Close Panel on Exit?"=w268:bool)
            n81 = Select(t="//UI: Front Panel State >> Close", s=w268, f="") -> (s? t:f=w265:string)
            n82 = call <vilib>:"Add State(s) to Queue__jki_lib_state_machine.vi"("State(s) in Front (\"\")"="USB4431: Shutdown\nData: Cleanup\nEvents: Unregister", "State(s) in (\"\")"="Process: Sync", "State(s) at Back (\"\")"="Exit") -> ("States Out"=w259:string)  [unwired: 12 in]
            n83 = call <vilib>:"Add State(s) to Queue__jki_lib_state_machine.vi"("State(s) in (\"\")"=w265, "State(s) at Back (\"\")"=w259) -> ("States Out"=w264:string)  [unwired: 13 in]
            n84 = call <vilib>:"Add State(s) to Queue__jki_lib_state_machine.vi"("State(s) in Front (\"\")"=w264, "State(s) in (\"\")"=w271) -> ("States Out"=w270:string)  [unwired: 13 in]
          }
          frame "---------- Process ----------" {
            # "Template Separator\n(You can make a copy of, or modify, this frame)"
            n85 = call <vilib>:"Add State(s) to Queue__jki_lib_state_machine.vi"("State(s) in (\"\")"=w276) -> ("States Out"=w275:string)  [unwired: 14 in]
          }
          frame "Process: Sync" {
            n86 = Unbundle By Name(w284) -> ("Core"=w280:T9)
            n87 = disable-structure shown="Enabled" {
              disable-tunnel: [w290 FALSE ("Don't run?")] -> w283
              disable-tunnel: w280 -> [_ _]
              disable-tunnel: w279 -> [w289 _]
              disable-tunnel: [w288 _] -> w278
              frame Enabled {
                n88 = call <vilib>:"WaitOnProcessSync.vi"("error in (no error)"=w289) -> ("error out"=w288:errorcluster, "Don't run?"=w290:bool)  [unwired: 8 in, 1 out]
              }
              frame Disabled {
              }
            }
            n89 = Select(t="Data: Cleanup\nEvents: Unregister\nExit", s=w283, f="") -> (s? t:f=w277:string)
            n90 = call <vilib>:"Add State(s) to Queue__jki_lib_state_machine.vi"("State(s) in Front (\"\")"=w277, "State(s) in (\"\")"=w287) -> ("States Out"=w286:string)  [unwired: 13 in]
          }
          frame "---------- Events ----------" {
            # "Template Separator\n(You can make a copy of, or modify, this frame)"
            n91 = call <vilib>:"Add State(s) to Queue__jki_lib_state_machine.vi"("State(s) in (\"\")"=w296) -> ("States Out"=w295:string)  [unwired: 14 in]
          }
          frame "Events: Register" {
            # "Expand to add\nmore events"
            # "Self Events (API Calls)"
            # "Base Class Protected Events"
            n92 = Unbundle By Name(w306) -> ("Self Reference"=w298:refnum<class "SynchiIO.PXI4461.lvclass">)
            n93 = call "SynchIO.USB4431.GetProtectedEvents.vi"("SynchIO.USB4431"=w298) -> ("Protected Events"=w304:T10, "SynchIO.USB4431 out"=w297:refnum<class "SynchIO.USB4431.lvclass">)  [unwired: 8 in, 1 out]
            n94 = call "SynchiIO.PXI4461.GetProtectedEvents.vi"("SynchiIO.PXI4461"=w297) -> ("error out"=w300:errorcluster, "Protected Events"=w299:T11)  [unwired: 8 in, 1 out]
            n95 = register-events(w299, w304) -> (reference out=w305:refnum<event-registration>, error out=w302:errorcluster)  [unwired: 2 in]
            n96 = Merge Errors(w303, w302, w300) -> (w301:errorcluster)  [unwired: 1 in]
            n97 = call <vilib>:"Add State(s) to Queue__jki_lib_state_machine.vi"("State(s) in (\"\")"=w308) -> ("States Out"=w307:string)  [unwired: 14 in]
          }
          frame "Events: Unregister" {
            n98 = Unregister For Events(event registration refnum=w311, error in=w310) -> (error out=w309:errorcluster)
            n99 = call <vilib>:"Clear Errors.vi"("error in (no error)"=w309) -> ()  [unwired: 5 in, 2 out]
            n100 = call <vilib>:"Add State(s) to Queue__jki_lib_state_machine.vi"("State(s) in (\"\")"=w314) -> ("States Out"=w313:string)  [unwired: 14 in]
          }
          frame "---------- API ----------" {
            n101 = call <vilib>:"Add State(s) to Queue__jki_lib_state_machine.vi"("State(s) in (\"\")"=w319) -> ("States Out"=w318:string)  [unwired: 14 in]
          }
          frame "API: NewData" {
            n102 = Unbundle By Name(w323) -> ("Your string data"=w320:string)  [unwired: 1 out]
            n103 = call "SynchIO.USB4431.SetData.vi"("error in (no error)"=w322, "Data In"=w320) -> ("error out"=w321:errorcluster)  [unwired: 8 in, 1 out]
            n104 = call <vilib>:"Add State(s) to Queue__jki_lib_state_machine.vi"("State(s) in (\"\")"=w326, "State(s) at Back (\"\")"=w320) -> ("States Out"=w325:string)  [unwired: 13 in]
          }
          frame "API: Initialize" {
            n105 = call <vilib>:"Add State(s) to Queue__jki_lib_state_machine.vi"("State(s) in (\"\")"=w331) -> ("States Out"=w330:string)  [unwired: 14 in]
          }
          frame "----------USB-4431---------- " {
            n106 = call <vilib>:"Add State(s) to Queue__jki_lib_state_machine.vi"("State(s) in (\"\")"=w336) -> ("States Out"=w335:string)  [unwired: 14 in]
          }
          frame "USB-4431: Initialize" {
            w338 = 10123 items=["Finite Samples"=10178, "Continuous Samples"=10123] ("sample mode")
            n107 = Unbundle By Name(w345) -> ("AI Buffer Size (S)"=w337:i32, "AI Configuration"=w349:T2, "AO Configuration"=w348:T3, "AO"=w347:T4, "sampling info"=w346:cluster{"Fs":dbl, "#s":dbl})
            n108 = call "4431 USB - Create IO Channels.vi"("sample mode"=w338, "error in"=w342, "AI Buffer Size (S)"=w337, "sampling info"=w346, "AO"=w347, "AO Configuration"=w348, "AI Configuration"=w349) -> ("AO Task"=w339:refnum<k21>[], "AI task"=w340:refnum<k21>[], "error out"=w341:errorcluster)  [unwired: 1 in, 1 out]
            n109 = Bundle By Name(cluster=w345, "AI task"=w340, "AO Task"=w339) -> (w344:T8)
            n110 = call <vilib>:"Add State(s) to Queue__jki_lib_state_machine.vi"("State(s) in Front (\"\")"="USB-4431: ReadWrite" ("message"), "State(s) in (\"\")"=w352) -> ("States Out"=w351:string)  [unwired: 13 in]
          }
          frame "USB-4431: ReadWrite" {
            n111 = Unbundle By Name(w366) -> ("AI task"=w359:refnum<k21>[], "AO Task"=w360:refnum<k21>[], "sampling info"=w364:cluster{"Fs":dbl, "#s":dbl}, "AO Data"=w358:waveform(dbl)[], "Iteration"=w353:i32)
            n112 = Equal To 0?(x=w353) -> (x = 0?=w355:bool)
            n113 = call "4461 - AI AND AI - Read AND Write Uneven -- Array.vi"("Reset"=w355, "AO Array"=w358, "error in (no error)"=w356, "sampling info"=w364, "AO Task"=w360, "AI task"=w359) -> ("error out"=w361:errorcluster, "Input Signals"=w363:waveform(dbl)[])  [unwired: 4 in]
            "Signals Graph" <- w363
            n114 = Increment(x=w353) -> (x+1=w354:i32)
            n115 = case shown="False" "stop" {
              tunnel: ["USB-4431: Publish" "USB-4431: Shutdown"] -> w362
              frame False {
              }
              frame True {
              }
            }
            n116 = Bundle By Name(cluster=w366, "AI Data"=w363, "Iteration"=w354) -> (w365:T8)
            n117 = call <vilib>:"Add State(s) to Queue__jki_lib_state_machine.vi"("State(s) in Front (\"\")"=w362, "State(s) in (\"\")"=w369) -> ("States Out"=w368:string)  [unwired: 13 in]
          }
          frame "USB-4431: Publish" {
            n118 = Unbundle By Name(w378) -> ("AI Data"=w372:waveform(dbl)[], "writer endpoint"=w374:refnum<k21>)
            n119 = shared-variable-write(w374, w372) -> (w373:refnum<k21>)  [unwired: 2 in, 2 out]
            n120 = Bundle By Name(cluster=w378, "AI Data"=w372, "writer endpoint"=w373) -> (w377:T8)
            n121 = call <vilib>:"Add State(s) to Queue__jki_lib_state_machine.vi"("State(s) in Front (\"\")"="USB-4431: ReadWrite", "State(s) in (\"\")"=w381) -> ("States Out"=w380:string)  [unwired: 13 in]
          }
          frame "USB-4431: Shutdown" {
            n122 = Unbundle By Name(w388) -> ("AI task"=w386:refnum<k21>[], "AO Task"=w385:refnum<k21>[], "writer endpoint"=w383:refnum<k21>)
            n123 = Build Array (concatenate)(w386, w385) -> (w384:refnum<k21>[])
            n124 = for {
              tunnel: [w396] -> w390
              tunnel: w389 -> [w395]
              tunnel: w384 -> [w394] mode=indexing
              n125 = flat-sequence {
                tunnel: [w401] -> w397
                tunnel: w395 -> [w400]
                tunnel: w394 -> [w399]
                tunnel: [w402] -> w398
                tunnel: w397 -> [w402]
                tunnel: w398 -> [w405]
                tunnel: [w404] -> w396
                frame #0 {
                  n126 = call <vilib>:"DAQmx Stop Task.vi"("task/channels in"=w399, "error in"=w400) -> ("task out"=w401:refnum<k21>)  [unwired: 12 in, 1 out]
                }
                frame #1 {
                  n127 = Wait (ms)(milliseconds to wait=u32 50) -> ()  [unwired: 1 out]
                }
                frame #2 {
                  n128 = call <vilib>:"DAQmx Clear Task.vi"("task in"=w405) -> ("error out"=w404:errorcluster)  [unwired: 14 in]
                }
                frame #3 {
                  n129 = Wait (ms)(milliseconds to wait=u32 50) -> ()  [unwired: 1 out]
                }
              }
            }
            n130 = Flush Stream(11:w383) -> (3:w382:refnum<k21>)  [unwired: 3 in, 2 out]
            n131 = Destroy Stream Endpoint(11:w382) -> ()  [unwired: 1 in, 1 out]
            n132 = call <vilib>:"Add State(s) to Queue__jki_lib_state_machine.vi"("State(s) in Front (\"\")"="Macro: Exit", "State(s) in (\"\")"=w393) -> ("States Out"=w392:string)  [unwired: 13 in]
          }
        }
        n133 = call "StateHistory.vi"("Current State in"=w16) -> ("Current State out"=→"Current State":string, "delimited string"=→"State History":string)  [unwired: 9 in]
      }
    }
    frame Error {
    }
  }
  n134 = call-parent "Process.vi"("error in"=w2, "SMO"=w1) -> ("error out"=w6:errorcluster, "SMO out"=→"SynchiIO.PXI4461 out":refnum<class "SynchiIO.PXI4461.lvclass">)  [unwired: 8 in]
  n135 = Merge Errors(w6, w3) -> (→"error out":errorcluster)
